vi "FlatToRichniswitch_grpc_GetChannelNameResponse.vi"(5 "OutputClusterType":T1, 11 "InputCluster":T2) -> (3 "OutputCluster":T1)   [LabVIEW 2021, in "NI Switch_client.lvlib"]
uses:
  NI Switch_client.lvlib
  niswitch_grpc_GetChannelNameResponse_Flat.ctl
  niswitch_grpc_GetChannelNameResponse.ctl
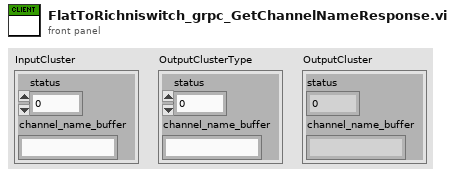
[diagram p1: front panel]
types:
  T1 = typedef "NI Switch_client.lvlib/niswitch_grpc_GetChannelNameResponse.ctl" = cluster{"status":i32, "channel_name_buffer":string}
  T2 = typedef "NI Switch_client.lvlib/niswitch_grpc_GetChannelNameResponse_Flat.ctl" = cluster{"status":i32, "channel_name_buffer":string}
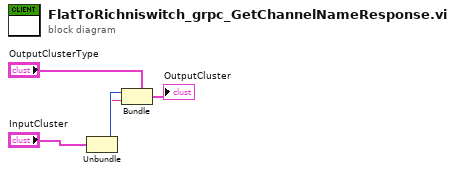
[diagram p0: block diagram]
diagram:
  n1 = Unbundle "Unbundle"("InputCluster") -> ("status"=w2:i32, "channel_name_buffer"=w1:string)
  n2 = Bundle "Bundle"(cluster="OutputClusterType", "status"=w2, "channel_name_buffer"=w1) -> (→"OutputCluster":T1)
